vi "Write ActorConfiguration.vi"(10 "ActorConfiguration":T1={"DeviceFamily"="", "BufferSize"=-1, "SyncDevice"=FALSE, "WriteData"=FALSE, "DeviceConfiguration"={"DeviceSpecificName"="MIPI_Camera", "HardwareReference"="PXIe-Slot2", "UsedResources"=[{"ResourceLocation"="FrontFacing", "ResourceData"=variant(string "Use this Variant to store your specific resource data.\nThis will be read from and written to with the JSON parsing API.\nIn the child implementation you can use the acessors provided to convert from the specific cluster to your own device's implementation")}]}}, 11 "Template in":refnum<class "Template.lvclass">) -> (3 "Template out":refnum<class "Template.lvclass">)   [LabVIEW 2020, in "Template.lvlib" / "Template.lvclass"]
uses:
  Template.lvclass
  typedefs/actor configuration.ctl
  typedefs/resource config/device configuration cluster.ctl
  typedefs/resource config/single resource cluster.ctl
  Template.lvclass/Template.ctl
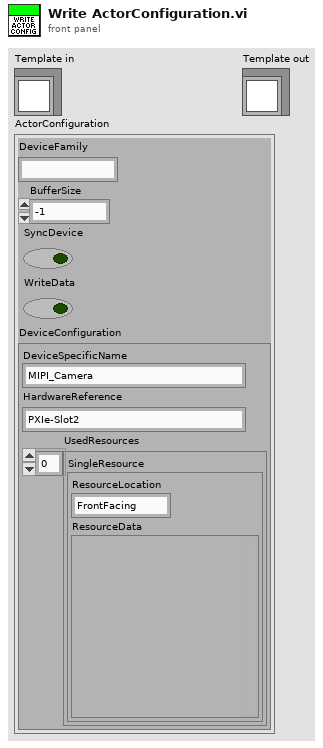
[diagram p1: front panel]
types:
  T1 = typedef "Template.lvlib/Template.lvclass/actor configuration.ctl" = cluster{"DeviceFamily":string, "BufferSize":i32, "SyncDevice":bool, "WriteData":bool, "DeviceConfiguration":T2}
  T2 = typedef "Template.lvlib/Template.lvclass/device configuration cluster.ctl" = cluster{"DeviceSpecificName":string, "HardwareReference":string, "UsedResources":T3[]}
  T3 = typedef "Template.lvlib/Template.lvclass/single resource cluster.ctl" = cluster{"ResourceLocation":string, "ResourceData":variant}
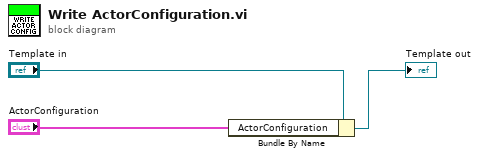
[diagram p0: block diagram]
diagram:
  n1 = Bundle By Name(cluster="Template in", "ActorConfiguration"="ActorConfiguration") -> (→"Template out":refnum<class "Template.lvclass">)
